vi "SerialSendHLcmd.vi"(0 "ASI stage":T1, 1 "Axis configuration":u16(ring) items=["No axis", "X", "Y", "Z", "XY", "XYZ"], 5 "Command":string, 7 "data in":cluster{"X in":dbl, "Y in":dbl, "Z in":dbl} {"Z in" format="%#.4f"; "Y in" format="%#.4f"; "X in" format="%#.4f"}, 11 "error in (no error)":errorcluster, 12 "Command type":enum16{"Query", "Where", "Imperative", "DU Y"}(ring)) -> (4 "Raw receive buffer":string, 6 "data out":cluster{"X out":dbl, "Y out":dbl, "Z out":dbl} {"Z out" format="%#.4f"; "Y out" format="%#.4f"; "X out" format="%#.4f"}, 15 "error out":errorcluster)   [LabVIEW 2010]
uses:
  stage properties.ctl
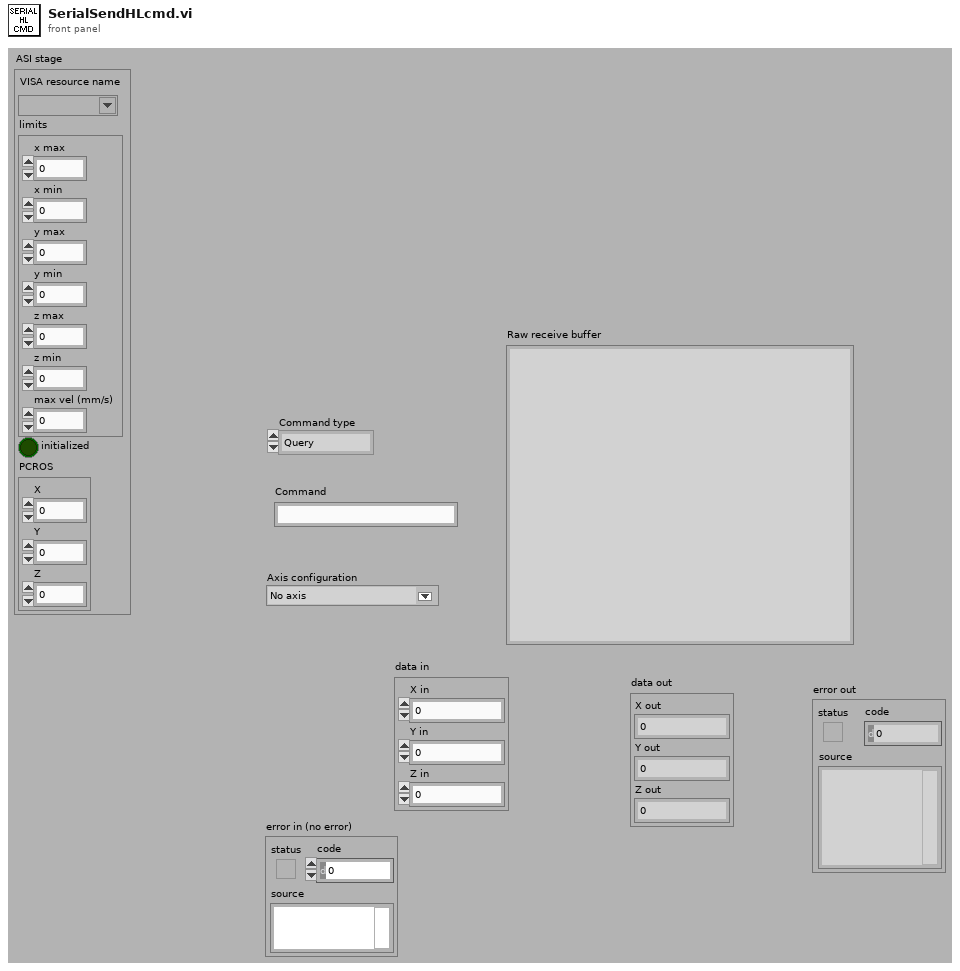
[diagram p1: front panel]
types:
  T1 = typedef "stage properties.ctl" = cluster{"VISA resource name":refnum<visa-resource-name>, "limits":cluster{"x max":dbl, "x min":dbl, "y max":dbl, "y min":dbl, "z max":dbl, "z min":dbl, "max vel (mm/s)":dbl}, "initialized":bool, "PCROS":cluster{"X":dbl, "Y":dbl, "Z":dbl}}
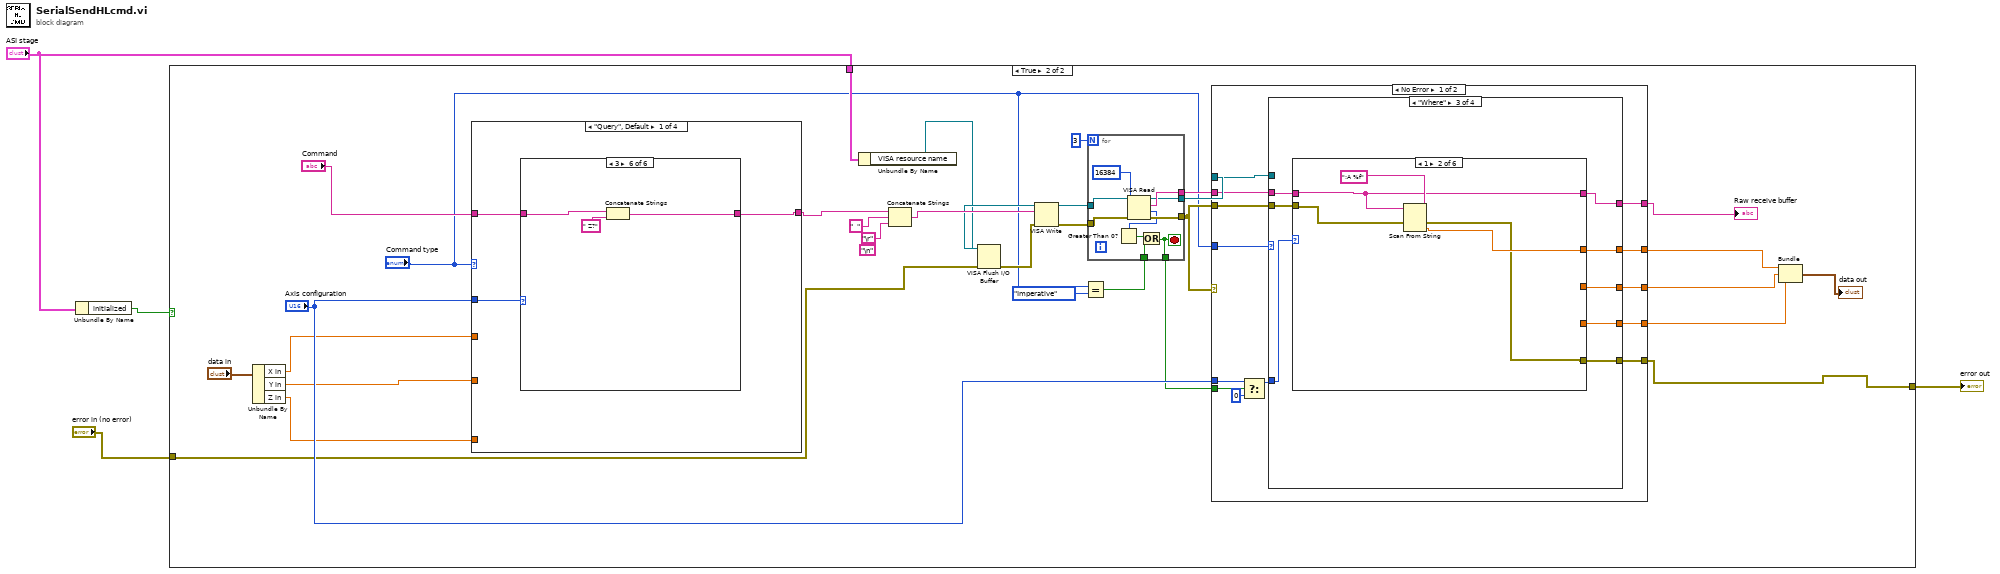
[diagram p0: block diagram]
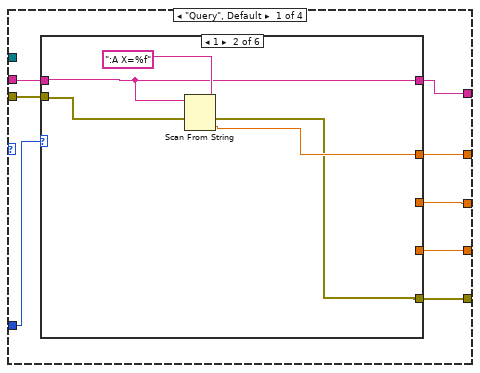
[diagram p3: hidden frame]
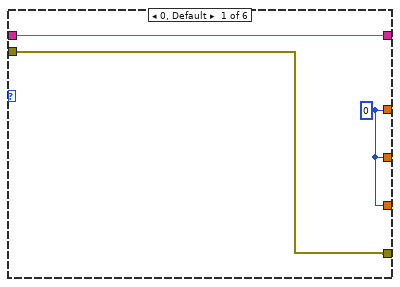
[diagram p4: hidden frame]
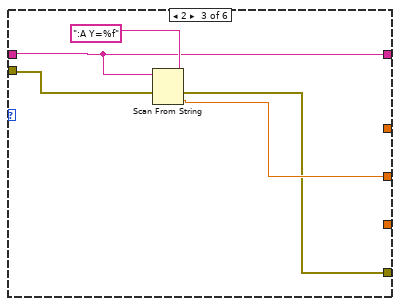
[diagram p5: hidden frame]
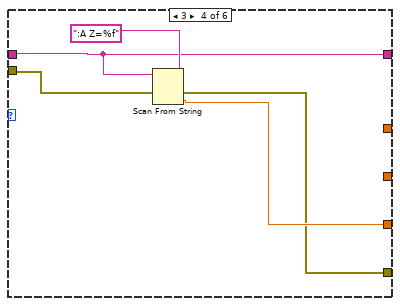
[diagram p6: hidden frame]
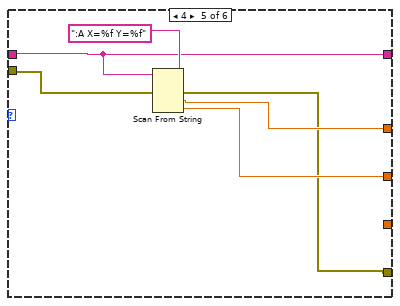
[diagram p7: hidden frame]
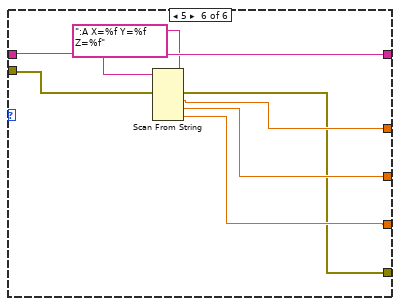
[diagram p8: hidden frame]
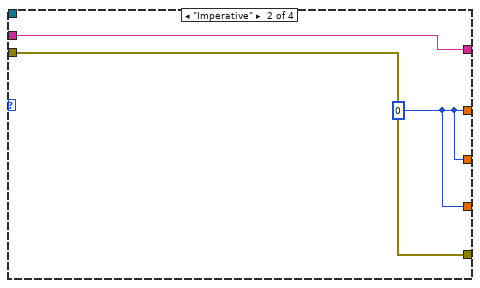
[diagram p9: hidden frame]
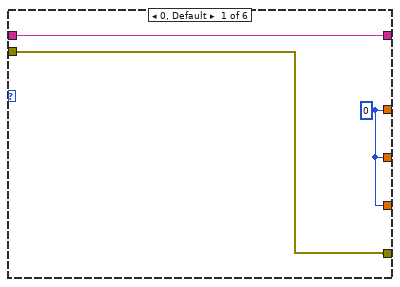
[diagram p10: hidden frame]
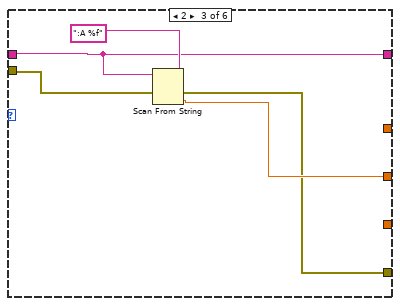
[diagram p11: hidden frame]
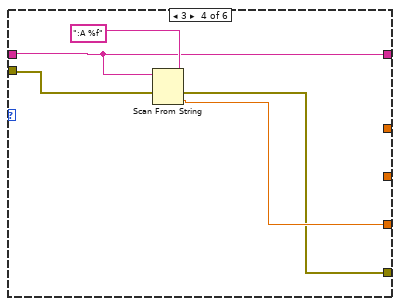
[diagram p12: hidden frame]
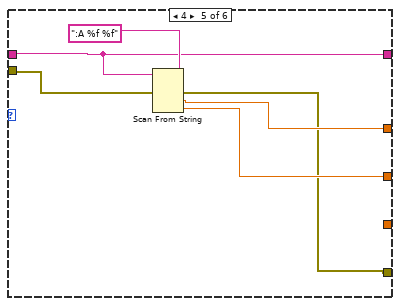
[diagram p13: hidden frame]
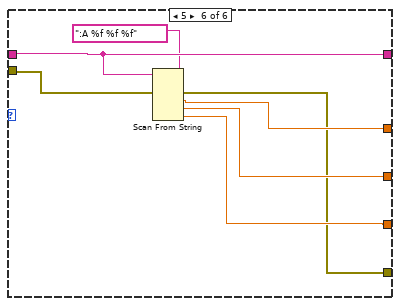
[diagram p14: hidden frame]
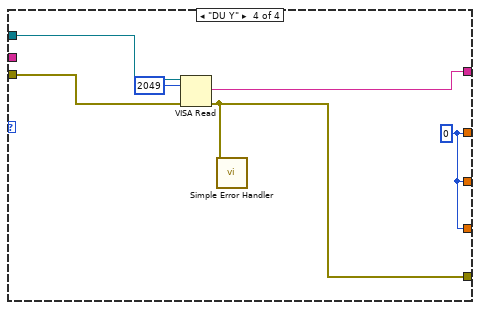
[diagram p15: hidden frame]
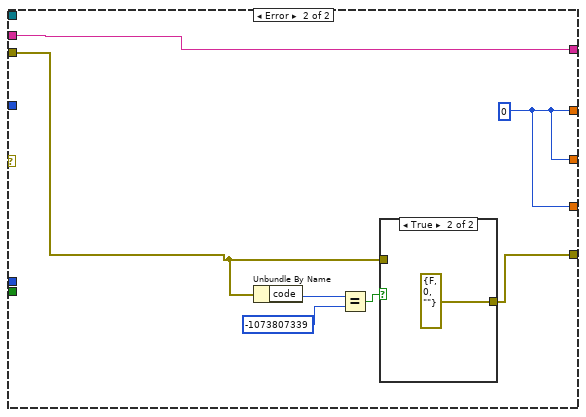
[diagram p16: hidden frame]
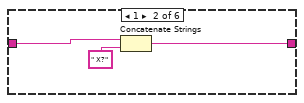
[diagram p19: hidden frame]
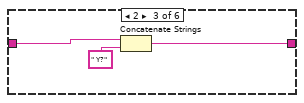
[diagram p20: hidden frame]
diagram:
  n1 = Unbundle By Name("ASI stage") -> ("initialized"=w1:bool)
  n2 = case shown="True" w1 {
    tunnel: "ASI stage" -> [_ w22]
    tunnel: [w5 w12] -> w4
    tunnel: "error in (no error)" -> [w5 w11]
    frame False {
    }
    frame True {
      (unwired) "\n"
      n3 = Unbundle By Name("data in") -> ("X in"=w20:dbl, "Y in"=w19:dbl, "Z in"=w18:dbl)
      n4 = case shown="\"Query\", Default" "Command type" {
        tunnel: "Command" -> [w157 w176 w199 _]
        tunnel: "Axis configuration" -> [w158 w177 w194 _]
        tunnel: w20 -> [_ _ w198 _]
        tunnel: w19 -> [_ _ w197 _]
        tunnel: w18 -> [_ _ w196 _]
        tunnel: [w156 w175 w195 "DU Y "] -> w36
        frame "Query", Default {
          n5 = case shown="3" w158 {
            tunnel: w157 -> [w159 w162 w165 w168 w171 w174]
            tunnel: [w159 w160 w163 w166 w169 w172] -> w156
            frame 0, Default {
            }
            frame 1 {
              n6 = Concatenate Strings "Concatenate Strings"(w162, " X?") -> (w160:string)
            }
            frame 2 {
              n7 = Concatenate Strings "Concatenate Strings"(w165, " Y?") -> (w163:string)
            }
            frame 4 {
              n8 = Concatenate Strings "Concatenate Strings"(w168, " X? Y?") -> (w166:string)
            }
            frame 5 {
              n9 = Concatenate Strings "Concatenate Strings"(w171, " X? Y? Z?") -> (w169:string)
            }
            frame 3 {
              n10 = Concatenate Strings "Concatenate Strings"(w174, " Z?") -> (w172:string)
            }
          }
        }
        frame "Where" {
          n11 = case shown="5" w177 {
            tunnel: w176 -> [w178 w181 w184 w187 w190 w193]
            tunnel: [w178 w179 w182 w185 w188 w191] -> w175
            frame 0, Default {
            }
            frame 1 {
              n12 = Concatenate Strings "Concatenate Strings"(w181, " X ") -> (w179:string)
            }
            frame 2 {
              n13 = Concatenate Strings "Concatenate Strings"(w184, " Y ") -> (w182:string)
            }
            frame 4 {
              n14 = Concatenate Strings "Concatenate Strings"(w187, " X Y") -> (w185:string)
            }
            frame 5 {
              n15 = Concatenate Strings "Concatenate Strings"(w190, " X Y Z ") -> (w188:string)
            }
            frame 3 {
              n16 = Concatenate Strings "Concatenate Strings"(w193, " Z") -> (w191:string)
            }
          }
        }
        frame "Imperative" {
          n17 = case shown="4" w194 {
            tunnel: w199 -> [w200 w204 w208 w212 w217 w223]
            tunnel: w198 -> [_ w202 _ _ w214 w220]
            tunnel: w197 -> [_ _ w205 _ w213 w219]
            tunnel: w196 -> [_ _ _ w209 _ w218]
            tunnel: [w200 w201 w206 w210 w215 w221] -> w195
            frame 0, Default {
            }
            frame 1 {
              n18 = Format Into String "Format Into String"(format string="  X=%7.4f", initial string=w204, w202) -> (resulting string=w201:string)  [unwired: 1 in, 1 out]
            }
            frame 2 {
              n19 = Format Into String "Format Into String"(format string="  Y=%7.4f", initial string=w208, w205) -> (resulting string=w206:string)  [unwired: 1 in, 1 out]
            }
            frame 3 {
              n20 = Format Into String "Format Into String"(format string=" Z=%7.4f", initial string=w212, w209) -> (resulting string=w210:string)  [unwired: 1 in, 1 out]
            }
            frame 4 {
              n21 = Format Into String "Format Into String"(format string=" X=%7.4f  Y=%7.4f", initial string=w217, w214, w213) -> (resulting string=w215:string)  [unwired: 1 in, 1 out]
            }
            frame 5 {
              n22 = Format Into String "Format Into String"(format string=" X=%7.4f  Y=%7.4f Z=%7.4f", initial string=w223, w220, w219, w218) -> (resulting string=w221:string)  [unwired: 1 in, 1 out]
            }
          }
        }
        frame "DU Y" {
        }
      }
      n23 = Unbundle By Name(w22) -> ("VISA resource name"=w13:refnum<visa-resource-name>)
      n24 = Concatenate Strings "Concatenate Strings"(w36, "  ", "\r") -> (w33:string)
      n25 = VISA Flush I/O Buffer(VISA resource name=w13, error in (no error)=w11) -> (VISA resource name out=w24:refnum<visa-resource-name>, error out=w32:errorcluster)  [unwired: 1 out]
      n26 = VISA Write(VISA resource name=w24, write buffer=w33, error in (no error)=w32) -> (VISA resource name out=w31:refnum<visa-resource-name>, error out=w30:errorcluster)  [unwired: 1 out]
      n27 = Equal?(x="Command type", y=enum16{"Query", "Where", "Imperative", "DU Y"}."Imperative") -> (x = y?=w7:bool)
      n28 = for {
        N: 3 -> [_]
        tunnel: w31 -> [w46]
        tunnel: w30 -> [w45]
        tunnel: [w44] -> w29
        tunnel: [w42] -> w26
        tunnel: [w41] -> w25
        tunnel: w7 -> [w38]
        tunnel: [w37] -> w6
        stop <- w37 stop-if-true
        n29 = VISA Read(VISA resource name=w46, byte count=u32 16384, error in (no error)=w45) -> (VISA resource name out=w41:refnum<visa-resource-name>, read buffer=w44:string, return count=w40:u32, error out=w42:errorcluster)
        n30 = Greater Than 0?(x=w40) -> (x > 0?=w39:bool)
        n31 = Or(x=w39, y=w38) -> (x .or. y?=w37:bool)
      }
      n32 = case shown="No Error" w26 {
        tunnel: w29 -> [w59 w152]
        tunnel: "Command type" -> [w58 _]
        tunnel: "Axis configuration" -> [w57 _]
        tunnel: [w56 w152] -> w27
        tunnel: [w55 w153] -> w17
        tunnel: [w54 w153] -> w16
        tunnel: [w53 w153] -> w15
        tunnel: w26 -> [w52 w147]
        tunnel: [w51 w149] -> w12
        tunnel: w25 -> [w50 _]
        tunnel: w6 -> [w48 _]
        frame No Error {
          n33 = Select(t=w57, s=w48, f=u16 0) -> (s? t:f=w49:u16)
          n34 = case shown="\"Where\"" w58 {
            tunnel: w59 -> [w66 w101 w108 _]
            tunnel: w49 -> [w67 _ w109 _]
            tunnel: [w65 w101 w107 w144] -> w56
            tunnel: [w63 w100 w105 w143] -> w55
            tunnel: [w62 w100 w104 w143] -> w54
            tunnel: [w61 w100 w103 w143] -> w53
            tunnel: w52 -> [w64 w99 w106 w145]
            tunnel: [w60 w99 w102 w141] -> w51
            tunnel: w50 -> [_ _ _ w146]
            frame "Query", Default {
              n35 = case shown="1" w67 {
                tunnel: w66 -> [w70 w74 w79 w84 w90 w98]
                tunnel: [w70 w74 w79 w84 w90 w98] -> w65
                tunnel: w64 -> [w68 w73 w78 w83 w89 w97]
                tunnel: [w69 w72 _ _ w88 w96] -> w63
                tunnel: [w69 _ w77 _ w87 w95] -> w62
                tunnel: [w69 _ _ w82 _ w93] -> w61
                tunnel: [w68 w71 w76 w81 w86 w92] -> w60
                frame 0, Default {
                  w69 = 0
                }
                frame 1 {
                  n36 = Scan From String "Scan From String"(format string=":A X=%f", input string=w74, error in=w73) -> (error out=w71:errorcluster, output 1=w72:dbl)  [unwired: 2 in, 2 out]
                }
                frame 2 {
                  n37 = Scan From String "Scan From String"(format string=":A Y=%f", input string=w79, error in=w78) -> (error out=w76:errorcluster, output 1=w77:dbl)  [unwired: 2 in, 2 out]
                }
                frame 3 {
                  n38 = Scan From String "Scan From String"(format string=":A Z=%f", input string=w84, error in=w83) -> (error out=w81:errorcluster, output 1=w82:dbl)  [unwired: 2 in, 2 out]
                }
                frame 4 {
                  n39 = Scan From String "Scan From String"(format string=":A X=%f Y=%f", input string=w90, error in=w89) -> (error out=w86:errorcluster, output 1=w88:dbl, output 2=w87:dbl)  [unwired: 3 in, 2 out]
                }
                frame 5 {
                  n40 = Scan From String "Scan From String"(format string=":A X=%f Y=%f Z=%f", input string=w98, error in=w97) -> (error out=w92:errorcluster, output 1=w96:dbl, output 2=w95:dbl, output 3=w93:dbl)  [unwired: 4 in, 2 out]
                }
              }
            }
            frame "Imperative" {
              w100 = 0
            }
            frame "Where" {
              n41 = case shown="1" w109 {
                tunnel: w108 -> [w112 w116 w121 w126 w132 w140]
                tunnel: [w112 w116 w121 w126 w132 w140] -> w107
                tunnel: w106 -> [w110 w115 w120 w125 w131 w139]
                tunnel: [w111 w114 _ _ w130 w138] -> w105
                tunnel: [w111 _ w119 _ w129 w137] -> w104
                tunnel: [w111 _ _ w124 _ w135] -> w103
                tunnel: [w110 w113 w118 w123 w128 w134] -> w102
                frame 0, Default {
                  w111 = 0
                }
                frame 1 {
                  n42 = Scan From String "Scan From String"(format string=":A %f", input string=w116, error in=w115) -> (error out=w113:errorcluster, output 1=w114:dbl)  [unwired: 2 in, 2 out]
                }
                frame 2 {
                  n43 = Scan From String "Scan From String"(format string=":A %f", input string=w121, error in=w120) -> (error out=w118:errorcluster, output 1=w119:dbl)  [unwired: 2 in, 2 out]
                }
                frame 3 {
                  n44 = Scan From String "Scan From String"(format string=":A %f", input string=w126, error in=w125) -> (error out=w123:errorcluster, output 1=w124:dbl)  [unwired: 2 in, 2 out]
                }
                frame 4 {
                  n45 = Scan From String "Scan From String"(format string=":A %f %f", input string=w132, error in=w131) -> (error out=w128:errorcluster, output 1=w130:dbl, output 2=w129:dbl)  [unwired: 3 in, 2 out]
                }
                frame 5 {
                  n46 = Scan From String "Scan From String"(format string=":A %f %f %f", input string=w140, error in=w139) -> (error out=w134:errorcluster, output 1=w138:dbl, output 2=w137:dbl, output 3=w135:dbl)  [unwired: 4 in, 2 out]
                }
              }
            }
            frame "DU Y" {
              w143 = 0
              n47 = VISA Read(VISA resource name=w146, byte count=u32 2049, error in (no error)=w145) -> (read buffer=w144:string, error out=w141:errorcluster)  [unwired: 2 out]
              n48 = call <vilib>:"Simple Error Handler.vi"("error in (no error)"=w141) -> ()  [unwired: 1 in, 8 out]
            }
          }
        }
        frame Error {
          w153 = 0
          n49 = Unbundle By Name(w147) -> ("code"=w151:i32)
          n50 = Equal?(x=w151, y=-1073807339) -> (x = y?=w148:bool)
          n51 = case shown="True" w148 {
            tunnel: [w154 errorcluster {"status"=FALSE, "code"=0, "source"=""}] -> w149
            tunnel: w147 -> [w154 _]
            frame False {
            }
            frame True {
            }
          }
        }
      }
      "Raw receive buffer" <- w27
      n52 = Bundle(w17, w16, w15) -> (→"data out":cluster{dbl, dbl, dbl})  [unwired: 1 in]
    }
  }
  "error out" <- w4
